vi "test-quintic-spline-03a.vi"() -> ()   [LabVIEW 2019]
uses:
  <vilib>/Rock Robotics/WPI/ThirdParty/JAS_Junk/TrajLib/POSEwCURVATURE.ctl
  <vilib>/Rock Robotics/WPI/ThirdParty/JAS_Junk/TrajLib/POSE2D.ctl
  <vilib>/Rock Robotics/WPI/ThirdParty/JAS_Junk/TrajLib/TRANSLATION2D.ctl
  <vilib>/Rock Robotics/WPI/ThirdParty/JAS_Junk/TrajLib/ROTATION2D.ctl
  <vilib>/Rock Robotics/WPI/ThirdParty/JAS_Junk/TrajLib/Rotation_CreateAngle.vi
  <vilib>/Rock Robotics/WPI/ThirdParty/JAS_Junk/TrajLib/Translation_Create.vi
  <vilib>/Rock Robotics/WPI/ThirdParty/JAS_Junk/TrajLib/Util_CalcDist.vi
  <vilib>/Rock Robotics/WPI/ThirdParty/JAS_Junk/TrajLib/Trajectory_Library.lvlib
panel:
  out "XY Graph":cluster{dbl[], dbl[]}(graph)
  out "Numb\nWaypoints":i32
  out "All Interior \nwayPoints\nFound (True)":bool
  out "end rot = 0":dbl
  out "end y = 0":dbl
  out "end x = 0":dbl
  out "start rot = 0":dbl
  out "start y = 0":dbl
  out "start x = 0":dbl
  out "max dtheta < 0.0872":dbl
  out "max dy < 0.00127":dbl
  out "max dx  < 0.127":dbl
  out "Overall Error":errorcluster
  out "Elements":i32
  out "Create Spline Error":errorcluster
  out "SplinePoses\nWCurve":T1[](array[typedef]) {"POSE"."ROTATION"."SIN" format="%13.4f"; "POSE"."ROTATION"."COS" format="%13.4f"; "POSE"."ROTATION"."VALUE" format="%13.4f"; "POSE"."TRANSLATION"."Y" format="%14.3f"; "POSE"."TRANSLATION"."X" format="%14.3f"}
  out "Elapsed Time":dbl
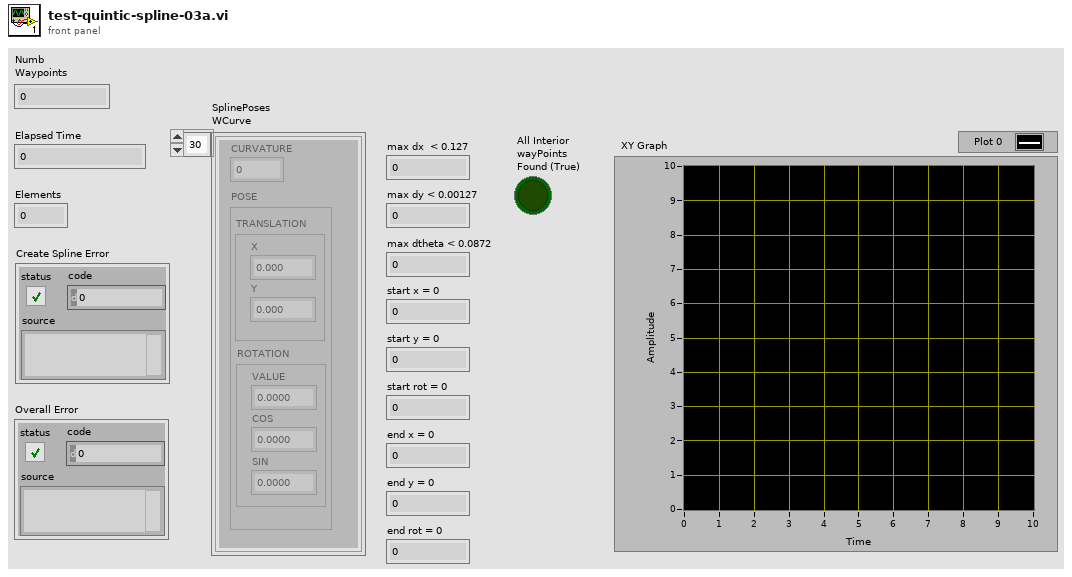
[diagram p1: front panel]
types:
  T1 = typedef "Trajectory_Library.lvlib/POSEwCURVATURE.ctl" = cluster{"CURVATURE":dbl, "POSE":T2}
  T2 = typedef "Trajectory_Library.lvlib/POSE2D.ctl" = cluster{"TRANSLATION":T3, "ROTATION":T4}
  T3 = typedef "Trajectory_Library.lvlib/TRANSLATION2D.ctl" = cluster{"X":dbl, "Y":dbl}
  T4 = typedef "Trajectory_Library.lvlib/ROTATION2D.ctl" = cluster{"VALUE":dbl, "COS":dbl, "SIN":dbl}
  T5 = typedef "Trajectory_Library.lvlib/SPLINE_CTRL_VECTOR.ctl" = cluster{"Xs":dbl[], "Ys":dbl[]}
  T6 = typedef "Trajectory_Library.lvlib/SPLINE.ctl" = cluster{"Degree":i32, "Coefficients":T7}
  T7 = typedef "NI_Matrix.lvlib/RealMatrix.ctl" = dbl[][]
  T8 = typedef "Trajectory_Library.lvlib/TWIST2D.ctl" = cluster{"dX":dbl, "dY":dbl, "dTHETA":dbl}
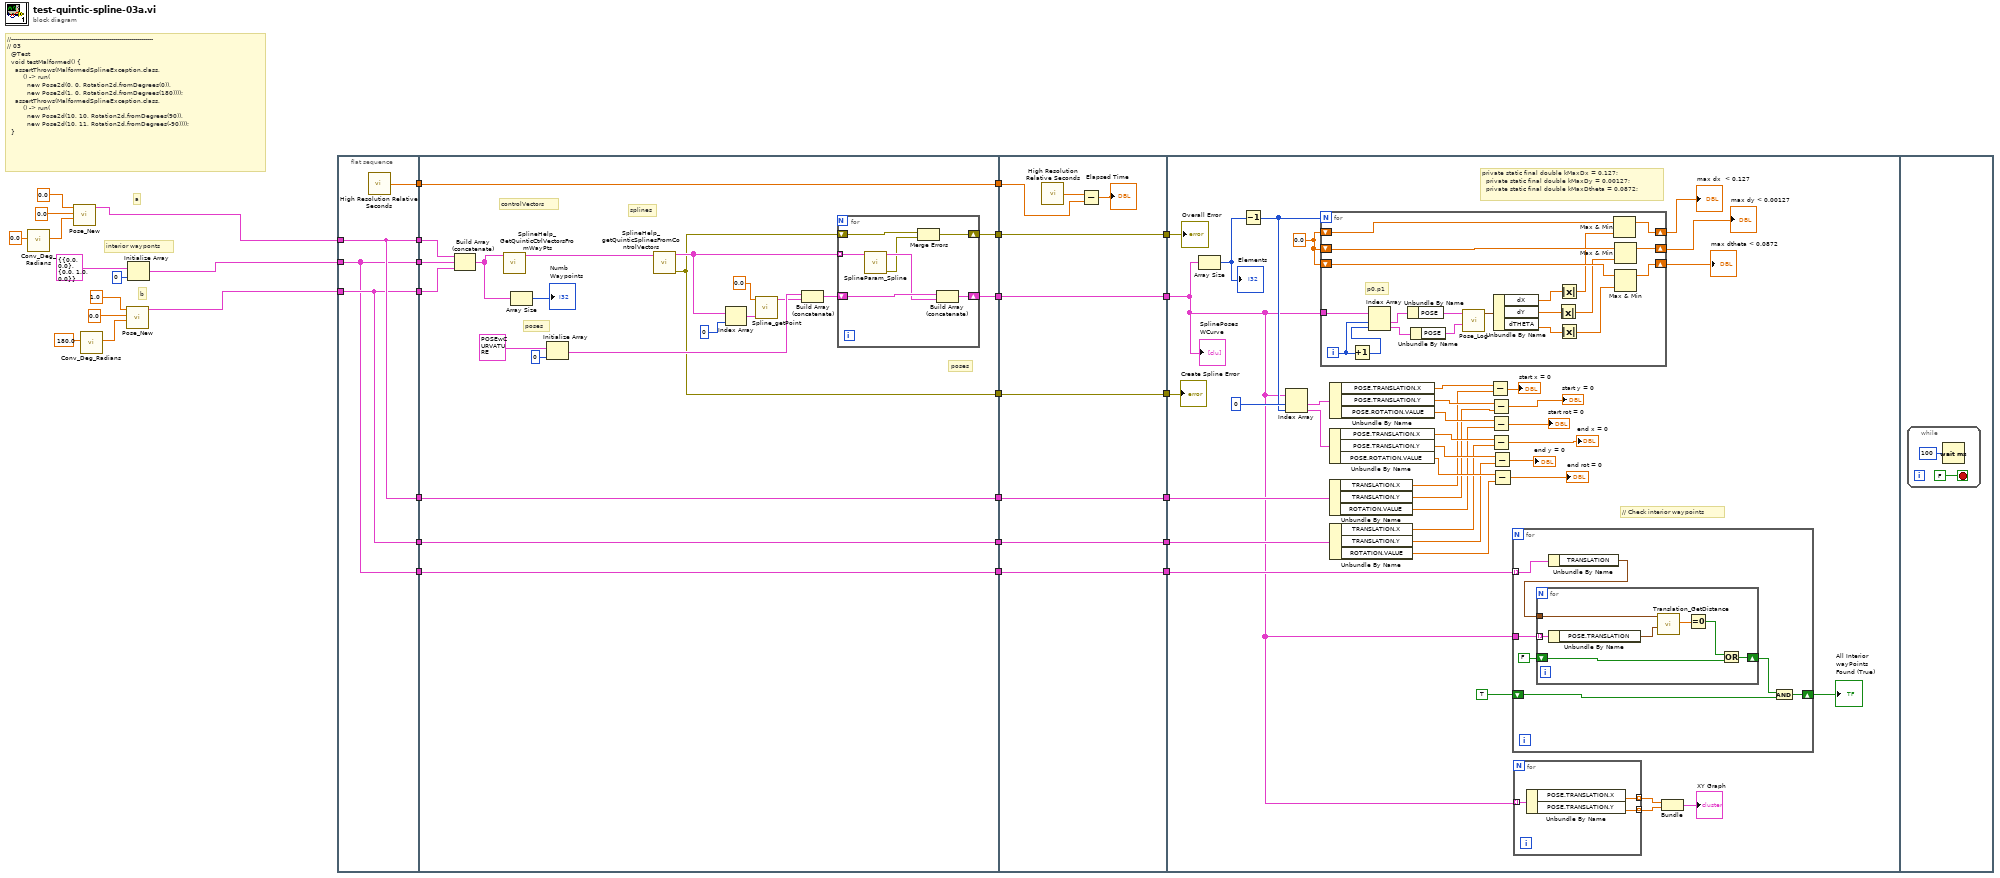
[diagram p0: block diagram]
diagram:
  # "interior wayponts"
  # "b"
  # "a"
  # "//-----------------------------------------------------------------------\n// 03\n  @Test\n  void testMalformed() {\n    assertThrows(MalformedSplineException.class,\n        () -> run(\n          new Pose2d(0, 0, Rotation2d.fromDegrees(0)),\n          new Pose2d(1, 0, Rotation2d.fromDegrees(180))));\n    assertThrows(MalformedSplineException.class,\n        () -> run(\n          new Pose2d(10, 10, Rotation2d.fromDegrees(90)),\n          new Pose2d(10, 11, Rotation2d.fromDegrees(-90))));\n  }"
  n1 = call <vilib>:"Conv_Deg_Radians.vi"("Degress"=0.0) -> ("Radians"=w4:dbl)  [unwired: 10 in]
  n2 = call <vilib>:"Pose_New.vi"("Heading"=w4, "Y"=0.0, "X"=0.0) -> ("out POSe"=w1:T2)  [unwired: 8 in]
  n3 = call <vilib>:"Conv_Deg_Radians.vi"("Degress"=180.0) -> ("Radians"=w7:dbl)  [unwired: 10 in]
  n4 = call <vilib>:"Pose_New.vi"("Heading"=w7, "Y"=0.0, "X"=1.0) -> ("out POSe"=w32:T2)  [unwired: 8 in]
  n5 = Initialize Array(T2 {"TRANSLATION"={"X"=0.0, "Y"=0.0}, "ROTATION"={"VALUE"=0.0, "COS"=1.0, "SIN"=0.0}} ("POSE"), 0 ("dimension size")) -> (w11:T2[])
  n6 = flat-sequence {
    tunnel: w1 -> [w36]
    tunnel: [w36] -> w33
    tunnel: w32 -> [w35]
    tunnel: [w35] -> w31
    tunnel: [w37] -> w30
    tunnel: [w36] -> w22
    tunnel: [w35] -> w19
    tunnel: [w34] -> w14
    tunnel: w11 -> [w34]
    tunnel: [w34] -> w10
    tunnel: w33 -> [w43]
    tunnel: w31 -> [w41]
    tunnel: [w59] -> w29
    tunnel: w30 -> [w59]
    tunnel: [w49] -> w28
    tunnel: [w48] -> w26
    tunnel: [w47] -> w24
    tunnel: w22 -> [w46]
    tunnel: [w46] -> w21
    tunnel: w19 -> [w45]
    tunnel: [w45] -> w18
    tunnel: [w44] -> w15
    tunnel: w14 -> [w44]
    tunnel: w10 -> [w40]
    tunnel: w29 -> [w75]
    tunnel: w28 -> [w74]
    tunnel: [w74] -> w27
    tunnel: w26 -> [w73]
    tunnel: [w73] -> w25
    tunnel: w24 -> [w72]
    tunnel: [w72] -> w23
    tunnel: w21 -> [w69]
    tunnel: [w69] -> w20
    tunnel: w18 -> [w68]
    tunnel: [w68] -> w17
    tunnel: [w67] -> w16
    tunnel: w15 -> [w67]
    tunnel: w27 -> [w77]
    tunnel: w25 -> [w113]
    tunnel: w23 -> [w112]
    tunnel: w20 -> [w106]
    tunnel: w17 -> [w105]
    tunnel: w16 -> [w82]
    frame #0 {
      n7 = call <vilib>:"High Resolution Relative Seconds.vi"() -> ("relative seconds"=w37:dbl)
    }
    frame #1 {
      # "poses"
      # "poses"
      # "splines"
      # "controlVectors"
      n8 = Build Array (concatenate)(w43, w40, w41) -> (w39:T2[])
      n9 = call <vilib>:"SplineHelp_GetQuinticCtrlVectorsFromWayPts.vi"("WayPoints"=w39) -> ("SplineControlVectors"=w42:T5[])  [unwired: 10 in]
      n10 = Array Size(array=w39) -> (size(s)=→"Numb\nWaypoints":i32)
      n11 = Initialize Array(T1 {"CURVATURE"=0.0, "POSE"={"TRANSLATION"={"X"=0.0, "Y"=0.0}, "ROTATION"={"VALUE"=0.0, "COS"=1.0, "SIN"=0.0}}} ("POSEwCURVATURE"), 0 ("dimension size")) -> (w53:T1[])
      n12 = call <vilib>:"SplineHelp_getQuinticSplinesFromControlVectors.vi"("ControlVectors"=w42) -> ("error out"=w48:errorcluster, "splines"=w50:T6[])  [unwired: 9 in]
      n13 = Index Array(array=w50, index=0) -> (element=w55:T6)
      n14 = call <vilib>:"Spline_getPoint.vi"("inputSPLINE"=w55, "Time"=0.0) -> ("POSEwCURVATURE"=w52:T1)  [unwired: 9 in]
      n15 = Build Array (concatenate)(w53, w52) -> (w51:T1[])
      n16 = for {
        shift-right: [w63] -> w49
        shift-left: w51 -> [w65]
        tunnel: w50 -> [w66] mode=indexing
        shift-right: [w61] -> w47
        shift-left: w48 -> [w62]
        n17 = call <vilib>:"SplineParam_Spline.vi"("inputSPLINE"=w66) -> ("error out"=w60:errorcluster, "outputPOSEwCURVATURE"=w64:T1[])  [unwired: 9 in]
        n18 = Merge Errors(w62, w60) -> (w61:errorcluster)
        n19 = Build Array (concatenate)(w65, w64) -> (w63:T1[])
      }
    }
    frame #2 {
      n20 = call <vilib>:"High Resolution Relative Seconds.vi"() -> ("relative seconds"=w70:dbl)
      n21 = Subtract(x=w70, y=w75) -> (x-y=→"Elapsed Time":dbl)
    }
    frame #3 {
      w110 = 0.0
      # "// Check interior waypoints"
      # "private static final double kMaxDx = 0.127;\n  private static final double kMaxDy = 0.00127;\n  private static final double kMaxDtheta = 0.0872;"
      n22 = Array Size(array=w77) -> (size(s)=w111:i32)
      "Elements" <- w111
      n23 = Decrement(x=w111) -> (x-1=w103:i32)
      n24 = Index Array(array=w77, index #1=0 ("index"), index #2=w103) -> (element #1=w102:T1, element #2=w101:T1)
      n25 = for {
        N: w103 -> [_]
        tunnel: w77 -> [w148]
        shift-right: [w139] -> w109
        shift-left: w110 -> [w136]
        shift-right: [w137] -> w107
        shift-left: w110 -> [w134]
        shift-right: [w138] -> w108
        shift-left: w110 -> [w135]
        i -> [w150]
        # "p0,p1"
        n26 = Increment(x=w150) -> (x+1=w149:i32)
        n27 = Index Array(array=w148, index #1=w150, index #2=w149) -> (element #1=w147:T1, element #2=w146:T1)
        n28 = Unbundle By Name(w147) -> ("POSE"=w145:T2)
        n29 = Unbundle By Name(w146) -> ("POSE"=w144:T2)
        n30 = call <vilib>:"Pose_Log.vi"("end POSE"=w144, "in POSE"=w145) -> ("out TWIST"=w143:T8)  [unwired: 9 in]
        n31 = Unbundle By Name(w143) -> ("dX"=w140:dbl, "dY"=w141:dbl, "dTHETA"=w142:dbl)
        n32 = Absolute Value(x=w141) -> (abs(x)=w132:dbl)
        n33 = Absolute Value(x=w140) -> (abs(x)=w133:dbl)
        n34 = Absolute Value(x=w142) -> (abs(x)=w131:dbl)
        n35 = Max & Min(x=w136, y=w133) -> (max(x,y)=w139:dbl)  [unwired: 1 out]
        n36 = Max & Min(x=w135, y=w132) -> (max(x,y)=w138:dbl)  [unwired: 1 out]
        n37 = Max & Min(x=w134, y=w131) -> (max(x,y)=w137:dbl)  [unwired: 1 out]
      }
      "max dx  < 0.127" <- w109
      "max dy < 0.00127" <- w108
      "max dtheta < 0.0872" <- w107
      n38 = Unbundle By Name(w101) -> ("POSE.TRANSLATION.X"=w97:dbl, "POSE.TRANSLATION.Y"=w96:dbl, "POSE.ROTATION.VALUE"=w95:dbl)
      n39 = Unbundle By Name(w106) -> ("TRANSLATION.X"=w94:dbl, "TRANSLATION.Y"=w93:dbl, "ROTATION.VALUE"=w92:dbl)
      n40 = Unbundle By Name(w102) -> ("POSE.TRANSLATION.X"=w100:dbl, "POSE.TRANSLATION.Y"=w99:dbl, "POSE.ROTATION.VALUE"=w98:dbl)
      n41 = Unbundle By Name(w105) -> ("TRANSLATION.X"=w91:dbl, "TRANSLATION.Y"=w90:dbl, "ROTATION.VALUE"=w89:dbl)
      n42 = Subtract(x=w100, y=w94) -> (x-y=→"start x = 0":dbl)
      n43 = Subtract(x=w99, y=w93) -> (x-y=→"start y = 0":dbl)
      n44 = Subtract(x=w98, y=w92) -> (x-y=→"start rot = 0":dbl)
      n45 = Subtract(x=w97, y=w91) -> (x-y=→"end x = 0":dbl)
      n46 = Subtract(x=w96, y=w90) -> (x-y=→"end y = 0":dbl)
      n47 = Subtract(x=w95, y=w89) -> (x-y=→"end rot = 0":dbl)
      n48 = for {
        tunnel: w82 -> [w118] mode=indexing
        tunnel: w77 -> [w123]
        shift-right: [w122] -> w80
        shift-left: TRUE -> [w121]
        n49 = Unbundle By Name(w118) -> ("TRANSLATION"=w117:T3)
        n50 = for {
          tunnel: w123 -> [w127] mode=indexing
          shift-right: [w130] -> w119
          shift-left: FALSE -> [w129]
          tunnel: w117 -> [w128]
          n51 = Unbundle By Name(w127) -> ("POSE.TRANSLATION"=w126:T3)
          n52 = call <vilib>:"Translation_GetDistance.vi"("other Translation"=w126, "In Translation"=w128) -> ("Distance"=w125:dbl)  [unwired: 9 in]
          n53 = Equal To 0?(x=w125) -> (x = 0?=w124:bool)
          n54 = Or(x=w124, y=w129) -> (x .or. y?=w130:bool)
        }
        n55 = And(x=w119, y=w121) -> (x .and. y?=w122:bool)
      }
      "All Interior \nwayPoints\nFound (True)" <- w80
      n56 = for {
        tunnel: [w116] -> w79 mode=indexing
        tunnel: [w115] -> w78 mode=indexing
        tunnel: w77 -> [w114] mode=indexing
        n57 = Unbundle By Name(w114) -> ("POSE.TRANSLATION.X"=w116:dbl, "POSE.TRANSLATION.Y"=w115:dbl)
      }
      n58 = Bundle(w79, w78) -> (→"XY Graph":cluster{dbl[], dbl[]})  [unwired: 1 in]
      "SplinePoses\nWCurve" <- w77
      "Create Spline Error" <- w113
      "Overall Error" <- w112
    }
    frame #4 {
      n59 = while {
        stop <- FALSE stop-if-true
        n60 = Wait (ms)(milliseconds to wait=u32 100) -> ()  [unwired: 1 out]
      }
    }
  }
